vi "to string.vi"(8 "error in":errorcluster, 11 "fixed channel configuration in":refnum<class "ThreePhasePLL configuration.lvclass">) -> (0 "error out":errorcluster, 1 "data":string, 2 "version":string, 3 "fixed channel configuration out":refnum<class "ThreePhasePLL configuration.lvclass">)   [LabVIEW 2017, in "ThreePhasePLL configuration.lvclass"]
doc: "Provides an interface for saving a module configuration to a file or other serialized data source. It is recommended that all children of this class store data in two sets--data required for its own initialization, and any data required for parent initialization--and that each implementation uses the <b>Call Parent Method</b> primitive to serialize parent information.\nNI Tag Bus Module Framework 1.0.3.43\nNI Systems Engineering"
uses:
  ThreePhasePLL configuration.lvclass
  ThreePhasePLL configuration.lvclass/ThreePhasePLL configuration.ctl
  <vilib>/NI/DCAF/Tag Editor Core/control module/configuration/control module configuration.lvclass
  <vilib>/NI/Configuration Framework/serializable configuration/NISE_CEF_serializable configuration.lvclass
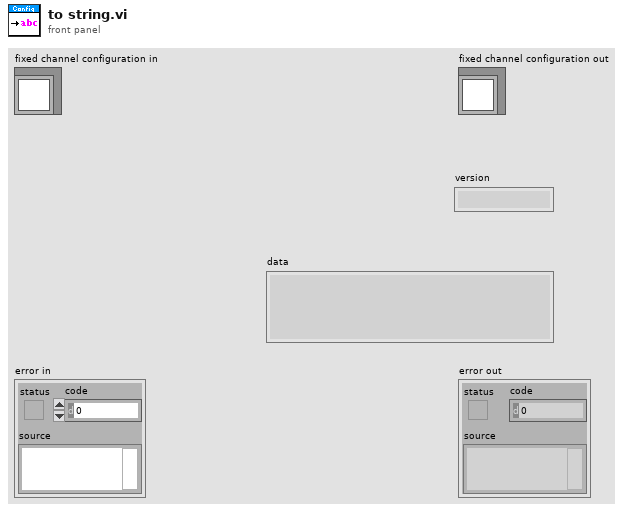
[diagram p1: front panel]
types:
  T1 = typedef "ThreePhasePLLInterface.lvlib/Configuration.ctl" = cluster{"PLLgains":T2, "PLLrange":T3, "dT":sgl, "expectedFreq":sgl, "lockDuration":sgl, "freqBoundaries":sgl}
  T2 = typedef "niFpgaPID_PIGains.ctl" = cluster{"proportional gain":sgl, "integral gain":sgl}
  T3 = typedef "niFpgaPID_OutputRange.ctl" = cluster{"output high (Inf)":sgl, "output low (-Inf)":sgl}
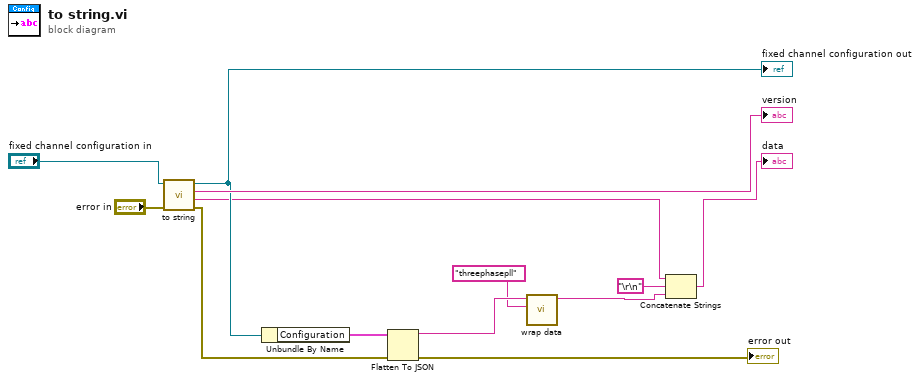
[diagram p0: block diagram]
diagram:
  n1 = call-parent "to string.vi"("error in"="error in", "fixed channel configuration in"="fixed channel configuration in") -> ("error out"=w4:errorcluster, "data"=w2:string, "version"=→"version":string, "fixed channel configuration out"=w5:refnum<class "ThreePhasePLL configuration.lvclass">)  [unwired: 6 in]
  "fixed channel configuration out" <- w5
  n2 = Unbundle By Name(w5) -> ("Configuration"=w9:T1)
  n3 = Flatten To JSON(anything=w9, error in (no error)=w4) -> (JSON string=w8:string, 11:→"error out":errorcluster)  [unwired: 1 in]
  n4 = call <vilib>:"wrap data.vi"("identifier"="threephasepll", "data to wrap"=w8) -> ("wrapped data"=w6:string)  [unwired: 9 in]
  n5 = Concatenate Strings(w2, "\r\n", w6) -> (→"data":string)
